vi "get crate map caen.vi"(0 "VISA in":refnum<visa-resource-name>, 3 "Crate":i32, 5 "error in":errorcluster) -> (14 "VISA out":refnum<visa-resource-name>, 16 "Crate Details":T1, 18 "Location Cluster out":T3, 19 "error out":errorcluster)   [LabVIEW 2018]
uses:
  location cluster.ctl
  crate.ctl
  card.ctl
  set location.ctl
  CAEN globals.vi
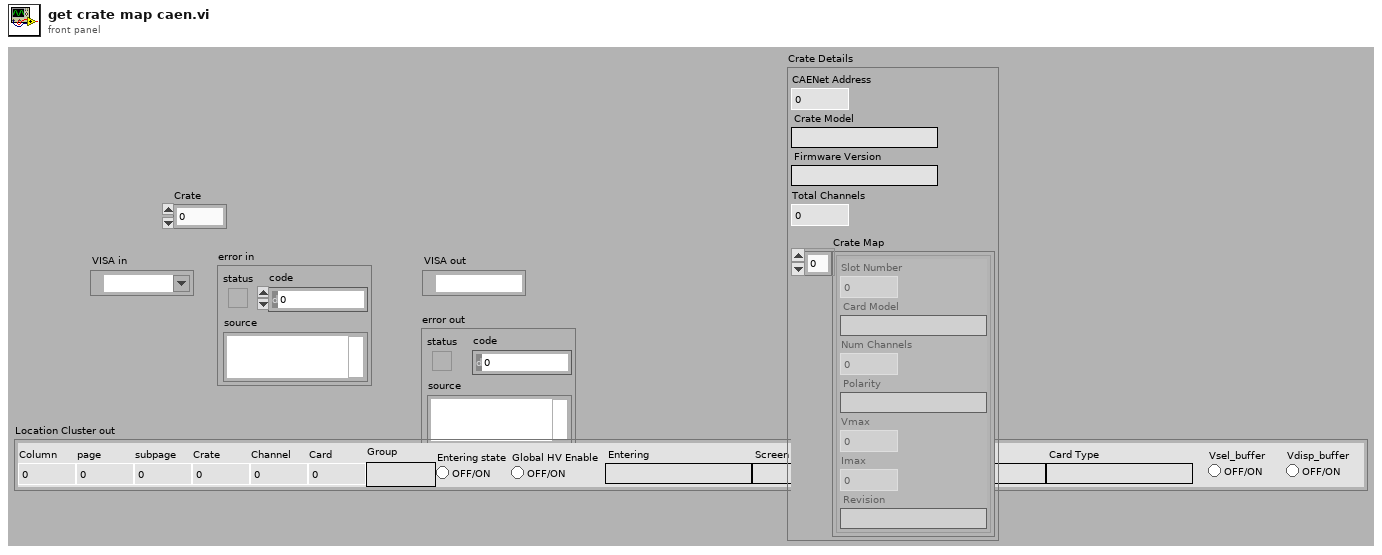
[diagram p1: front panel]
types:
  T1 = typedef "crate.ctl" = cluster{"CAENet Address":i32, "Crate Model":string, "Firmware Version":string, "Crate Map":T2[], "Total Channels":i32}
  T2 = typedef "card.ctl" = cluster{"Slot Number":i32, "Card Model":string, "Num Channels":i32, "Polarity":string, "Vmax":dbl, "Imax":dbl, "Revision":string}
  T3 = typedef "location cluster.ctl" = cluster{"Column":i32, "Card Type":string, "Channel":i32, "Card":i32, "Default response":string, "Entering":string, "Entering state":bool, "subpage":i32, "page":i32, "Crate":i32, "Screen":string, "Group":string, "Global HV Enable":bool, "Vsel_buffer":bool, "Vdisp_buffer":bool}
  T4 = typedef "set location.ctl" = cluster{"set index":i32, "set Screen":string, "set subpage":i32, "set column":i32, "Group":string, "Crate":i32}
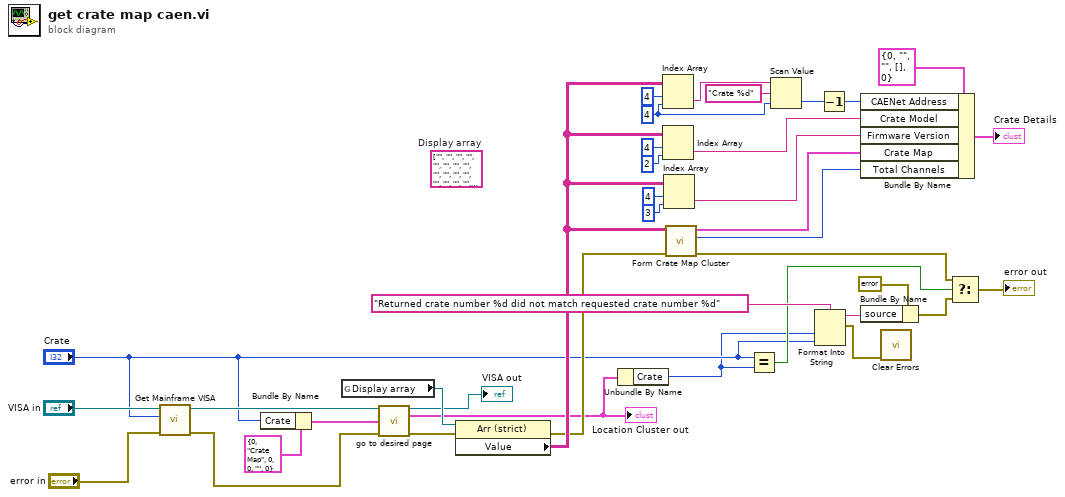
[diagram p0: block diagram]
diagram:
  (unwired) string[][] [["", "", "", "", "", ""], ["", "", "", "", "", ""], ["", "", "", "", "", ""], ["", "", "", "", "", ""], ["", "C.A.E.N.", "SY527", "V3.18", "Crate 01", ""], ["", "", "", "", "", ""], ["", "", "", "", "", ""], ["", "Crate map", "", "", "", ""], ["", "", "", "", "", ""], ["", "", "", "", "", ""], [" Slot 0:", "Mod. A734", "16 CH POSITIVE", "3000V", "3000.00uA --- Ser.", "6, Rel. 1.01"], [" Slot 1:", "Mod. A734", "16 CH POSITIVE", "3000V", "3000.00uA --- Ser.", "20, Rel. 1.01"], [" Slot 2:", "Mod. A734", "16 CH POSITIVE", "3000V", "3000.00uA --- Ser. 190, Rel. 1.01", ""], [" Slot 3:", "Mod. A734", "16 CH POSITIVE", "3000V", "3000.00uA --- Ser.", "13, Rel. 1.01"], [" Slot 4:", "Mod. A734", "16 CH POSITIVE", "3000V", "3000.00uA --- Ser.", "14, Rel. 1.01"], [" Slot 5:", "Mod. A734", "16 CH POSITIVE", "3000V", "3000.00uA --- Ser. 189, Rel. 1.01", ""], [" Slot 6:", "Mod. A734", "16 CH POSITIVE", "3000V", "3000.00uA --- Ser. 185, Rel. 1.01", ""], [" Slot 7:", "Not Present", "", "", "", ""], [" Slot 8:", "Mod. A938A", "25 CH NEGATIVE", "2200V", "1.20mA --- Ser.", "46, Rel. 1.01"], [" Slot 9:", "Mod. A938A", "25 CH NEGATIVE", "2200V", "1.20mA --- Ser.", "52, Rel. 1.01"], ["", "", "", "", "", ""], ["", "", "", "", "", ""], ["", "", "", "", "", ""], ["Press any key to continue", "", "", "", "", ""]]  # Display array
  w31 = 4 ("index (row)")
  n1 = call "Get Mainframe VISA.vi"("Error In"="error in", "Crate"="Crate", "VISA In"="VISA in") -> ("Error Out"=w2:errorcluster, "VISA out"=w5:refnum<visa-resource-name>)  [unwired: 6 in, 1 out]
  n2 = Bundle By Name(cluster=T4 {"set index"=0, "set Screen"="Crate Map", "set subpage"=0, "set column"=0, "Group"="", "Crate"=0} ("Set Cluster"), "Crate"="Crate") -> (w19:T4)
  n3 = global read "CAEN globals.vi" "Display array"() -> (w25:refnum<vi>)
  n4 = call "go to desired page.vi"("VISA in"=w5, "Set Cluster"=w19, "error in"=w2) -> ("VISA out"=→"VISA out":refnum<visa-resource-name>, "Location Cluster out"=w18:T3, "error out"=w23:errorcluster)  [unwired: 9 in, 1 out]
  "Location Cluster out" <- w18
  n5 = property class="Arr (strict)"(reference=w25, error in=w23) -> (error out=w22:errorcluster, "Value"=w24:string[][])  [unwired: 1 out]
  n6 = Unbundle By Name(w18) -> ("Crate"=w1:i32)
  n7 = Index Array(array=w24, index (row)=4, index (col)=w31) -> (element=w33:string)
  n8 = Index Array(array=w24, index (row)=4, index (col)=2 ("index (row)")) -> (element=w30:string)
  n9 = Index Array(array=w24, index (row)=4, index (col)=3 ("index (row)")) -> (element=w29:string)
  n10 = call "Form Crate Map Cluster.vi"("error in"=w22, "Display array"=w24) -> ("error out"=w7:errorcluster, "total channels"=w15:i32, "Card Map"=w28:T2[])  [unwired: 7 in]
  n11 = Equal?(x="Crate", y=w1) -> (x = y?=w8:bool)
  n12 = Scan Value(string=w33, format string="Crate %d", default (0 dbl)=w31) -> (value=w17:i32)  [unwired: 1 out]
  n13 = Format Into String(format string="Returned crate number %d did not match requested crate number %d" ("source"), w1, "Crate") -> (resulting string=w12:string, error out=w11:errorcluster)  [unwired: 2 in]
  n14 = Decrement(x=w17) -> (x-1=w16:i32)
  n15 = Bundle By Name(cluster=T1 {"CAENet Address"=0, "Crate Model"="", "Firmware Version"="", "Crate Map"=[], "Total Channels"=0} ("output cluster"), "CAENet Address"=w16, "Crate Model"=w30, "Firmware Version"=w29, "Crate Map"=w28, "Total Channels"=w15) -> (→"Crate Details":T1)
  n16 = Bundle By Name(cluster=errorcluster {"status"=TRUE, "code"=0, "source"=""} ("error out"), "source"=w12) -> (w10:errorcluster)
  n17 = call <vilib>:"Clear Errors.vi"("error in (no error)"=w11) -> ()  [unwired: 5 in, 2 out]
  n18 = Select(t=w7, s=w8, f=w10) -> (s? t:f=→"error out":errorcluster)
